vi "condition_control_array_v02.vi"(8 "error in":errorcluster, 11 "control array in":refnum<vi>[](array[refnum])) -> (0 "error out":errorcluster, 3 "control array out":refnum<vi>[](array[refnum]))   [LabVIEW 2019]
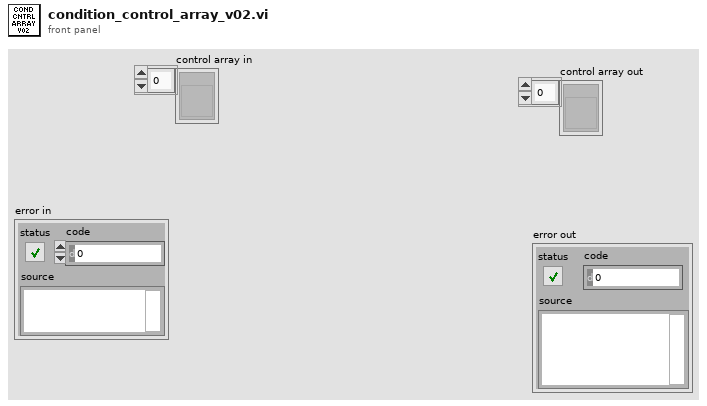
[diagram p1: front panel]
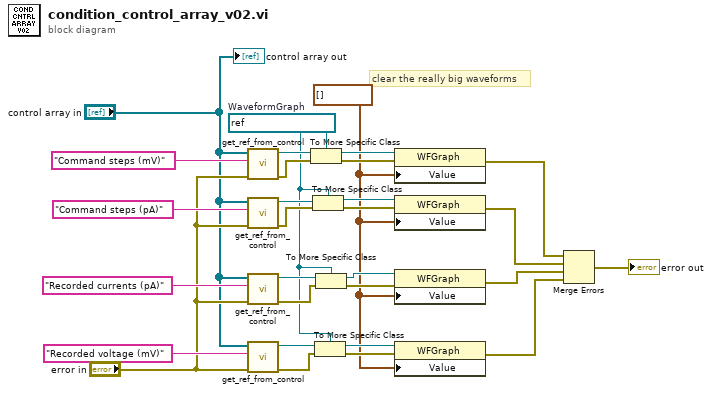
[diagram p0: block diagram]
diagram:
  w1 = waveform(dbl)[] []
  w2 = refnum<vi> refnum  # WaveformGraph
  # "clear the really big waveforms"
  n1 = call "get_ref_from_control.vi"("error in"="error in", "control label"="Command steps (mV)", "controls array"="control array in") -> ("error out"=w25:errorcluster, "reference out"=w24:refnum<vi>)  [unwired: 7 in]
  n2 = call "get_ref_from_control.vi"("error in"="error in", "control label"="Command steps (pA)", "controls array"="control array in") -> ("error out"=w19:errorcluster, "reference out"=w22:refnum<vi>)  [unwired: 7 in]
  n3 = call "get_ref_from_control.vi"("error in"="error in", "control label"="Recorded currents (pA)", "controls array"="control array in") -> ("error out"=w18:errorcluster, "reference out"=w21:refnum<vi>)  [unwired: 7 in]
  n4 = call "get_ref_from_control.vi"("error in"="error in", "control label"="Recorded voltage (mV)", "controls array"="control array in") -> ("error out"=w17:errorcluster, "reference out"=w20:refnum<vi>)  [unwired: 7 in]
  n5 = To More Specific Class(target class=w2, reference=w24, error in=w25) -> (specific class reference=w23:refnum<vi>, error out=w16:errorcluster)
  n6 = To More Specific Class(target class=w2, reference=w22, error in=w19) -> (specific class reference=w15:refnum<vi>, error out=w12:errorcluster)
  n7 = To More Specific Class(target class=w2, reference=w20, error in=w17) -> (specific class reference=w11:refnum<vi>, error out=w10:errorcluster)
  n8 = To More Specific Class(target class=w2, reference=w21, error in=w18) -> (specific class reference=w14:refnum<vi>, error out=w13:errorcluster)
  n9 = property class="WFGraph"(reference=w23, error in=w16, "Value"=w1) -> (error out=w9:errorcluster)  [unwired: 1 out]
  n10 = property class="WFGraph"(reference=w15, error in=w12, "Value"=w1) -> (error out=w8:errorcluster)  [unwired: 1 out]
  n11 = property class="WFGraph"(reference=w14, error in=w13, "Value"=w1) -> (error out=w7:errorcluster)  [unwired: 1 out]
  n12 = property class="WFGraph"(reference=w11, error in=w10, "Value"=w1) -> (error out=w6:errorcluster)  [unwired: 1 out]
  n13 = Merge Errors(w9, w8, w7, w6) -> (→"error out":errorcluster)
  "control array out" <- "control array in"
